vi "Backslash Codes to Normal String.vi"(11 "Backslash String in":string) -> (3 "Normal String out":string)   [LabVIEW 2018, in "String Data Type.lvclass"]
uses:
  String Data Type.lvclass
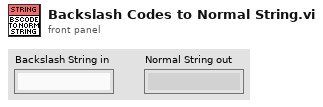
[diagram p1: front panel]
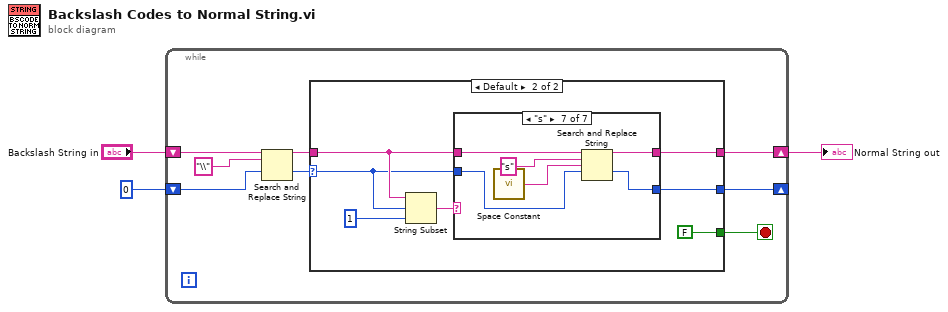
[diagram p0: block diagram]
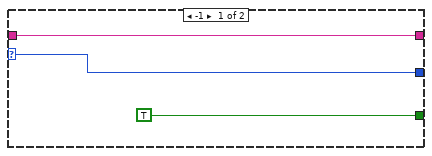
[diagram p2: hidden frame]
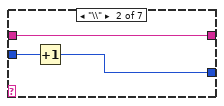
[diagram p4: hidden frame]
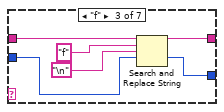
[diagram p5: hidden frame]
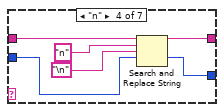
[diagram p6: hidden frame]
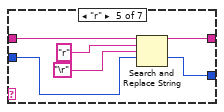
[diagram p7: hidden frame]
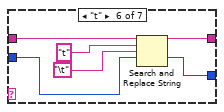
[diagram p8: hidden frame]
diagram:
  n1 = while {
    shift-right: [w5] -> _
    shift-left: 0 -> [w9]
    shift-right: [w4] -> w1
    shift-left: "Backslash String in" -> [w11]
    stop <- w6 stop-if-true
    n2 = Search and Replace String(input string=w11, search string="\\", offset=w9) -> (result string=w7:string, offset past replacement=w8:i32)  [unwired: 5 in, 2 out]
    n3 = case shown="Default" w8 {
      selector: w8 -> [w13 w18]
      tunnel: w7 -> [w12 w19]
      tunnel: [TRUE FALSE] -> w6
      tunnel: [w13 w17] -> w5
      tunnel: [w12 w16] -> w4
      frame -1 {
      }
      frame Default {
        n4 = String Subset(string=w19, offset (0)=w18, length (rest)=1 ("length (rest)")) -> (substring=w20:string)
        n5 = case shown="\"s\"" w20 {
          tunnel: w19 -> [w23 w26 w32 w38 w44 w50 w56]
          tunnel: w18 -> [w22 w25 w29 w35 w41 w47 w53]
          tunnel: [w22 w24 w28 w34 w40 w46 w52] -> w17
          tunnel: [w23 w26 w27 w33 w39 w45 w51] -> w16
          frame Default {
          }
          frame "\\" {
            n6 = Increment(x=w25) -> (x+1=w24:i32)
          }
          frame "f" {
            n7 = Search and Replace String(input string=w32, search string="f", replace string="\n", offset=w29) -> (result string=w27:string, offset past replacement=w28:i32)  [unwired: 4 in, 2 out]
          }
          frame "n" {
            n8 = Search and Replace String(input string=w38, search string="n", replace string="\n", offset=w35) -> (result string=w33:string, offset past replacement=w34:i32)  [unwired: 4 in, 2 out]
          }
          frame "r" {
            n9 = Search and Replace String(input string=w44, search string="r", replace string="\r", offset=w41) -> (result string=w39:string, offset past replacement=w40:i32)  [unwired: 4 in, 2 out]
          }
          frame "t" {
            n10 = Search and Replace String(input string=w50, search string="t", replace string="\t", offset=w47) -> (result string=w45:string, offset past replacement=w46:i32)  [unwired: 4 in, 2 out]
          }
          frame "s" {
            n11 = call <vilib>:"Space Constant.vi"() -> ("String"=w55:string)
            n12 = Search and Replace String(input string=w56, search string="s", replace string=w55, offset=w53) -> (result string=w51:string, offset past replacement=w52:i32)  [unwired: 4 in, 2 out]
          }
        }
      }
    }
  }
  "Normal String out" <- w1
